vi "Delete Project Item.vi"(7 "Type":string, 8 "error in (no error)":errorcluster, 9 "Item Name":string, 10 "Target Name":string, 11 "Project Sync Tools in":refnum<class "Project Sync Tools.lvclass">) -> (0 "error out":errorcluster, 3 "Project Sync Tools out":refnum<class "Project Sync Tools.lvclass">)   [LabVIEW 2019, in "Project Sync Tools.lvclass"]
uses:
  Project Sync Tools.lvclass
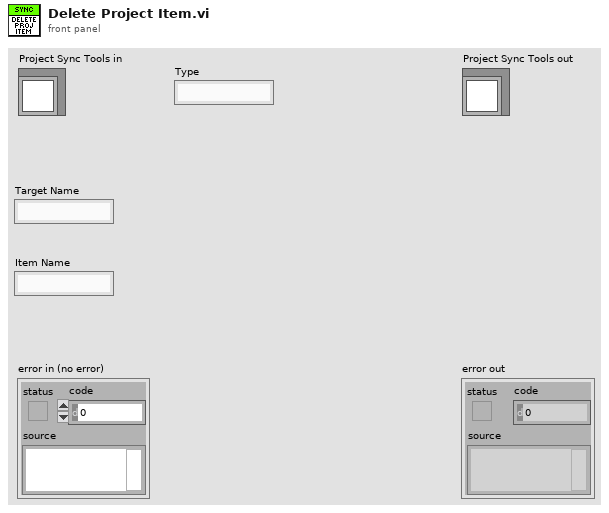
[diagram p1: front panel]
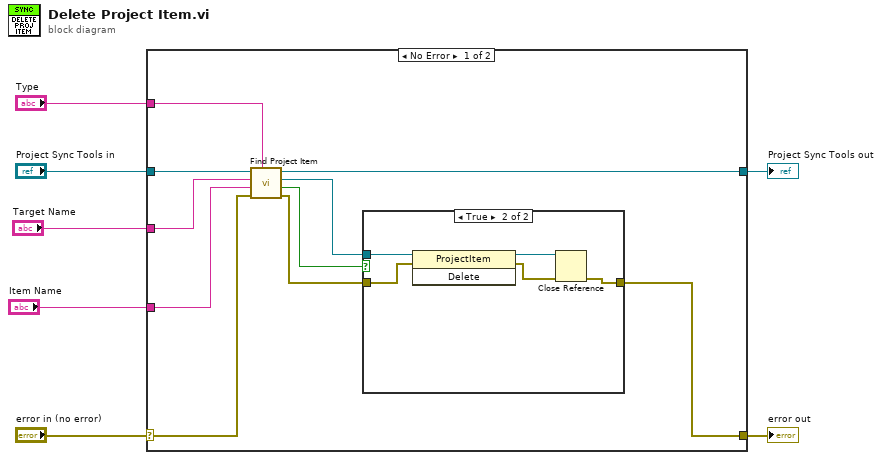
[diagram p0: block diagram]
diagram:
  n1 = case shown="No Error" "error in (no error)" {
    selector: "error in (no error)" -> [w12 w25]
    tunnel: [w8 w25] -> w6
    tunnel: [w16 w24] -> w4
    tunnel: "Project Sync Tools in" -> [w17 w24]
    tunnel: "Type" -> [w15 _]
    tunnel: "Target Name" -> [w14 _]
    tunnel: "Item Name" -> [w13 _]
    frame No Error {
      n2 = call "Find Project Item.vi"("Type"=w15, "error in (no error)"=w12, "Item Name"=w13, "Target Name"=w14, "Project Sync Tools in"=w17) -> ("error out"=w11:errorcluster, "Found ?"=w9:bool, "ProjectItem out"=w10:refnum<vi>, "Project Sync Tools out"=w16:refnum<class "Project Sync Tools.lvclass">)  [unwired: 3 in]
      n3 = case shown="True" w9 {
        tunnel: w11 -> [w18 w23]
        tunnel: w10 -> [_ w22]
        tunnel: [w18 w19] -> w8
        frame False {
        }
        frame True {
          n4 = invoke class="ProjectItem" method="Delete"(reference=w22, error in=w23) -> (reference out=w20:refnum<vi>, error out=w21:errorcluster)  [unwired: 1 in, 1 out]
          n5 = Close Reference(reference=w20, error in (no error)=w21) -> (error out=w19:errorcluster)
        }
      }
    }
    frame Error {
    }
  }
  "error out" <- w6
  "Project Sync Tools out" <- w4
